vi "Fit Mutiple Cernox Files.vi"() -> ()   [LabVIEW 2025]
panel:
  out "avg T":dbl[](array[numeric])
  out "Calculated T out":dbl[][](array[numeric])
  in  "Calculate R in":dbl[](array[numeric])=[70.34796, 80.267567, 85.278681, 91.166987, 98.217159]
  out "Linear Graph":cluster{dbl[], dbl[]}[](graph)
  out "Difference":cluster{dbl[], dbl[]}[](graph)
  in  "Polynomial order":i32=18
  in  "fit mode":T1(ring)=enum."LogT-1/R"
  in  "error in":errorcluster
  in  "Sources":T2(array[cluster])=[{"File Path"=path "\\\\myhome\\NHMFLDATA/Data/PPMS/October_2025/102425/m001_164026_102425.tdms", "offset (0)"=3810, "count (-1: all)"=39060, "channel name(s) in"=["LakeShore 336 (12) A", "LakeShore 336 (12) B Raw"], "group"="p"}, {"File Path"=path "\\\\myhome\\NHMFLDATA/Data/PPMS/October_2025/102225/m003_162726_102225.tdms", "offset (0)"=134648, "count (-1: all)"=-1, "channel name(s) in"=["LakeShore 336 (12) A", "LakeShore 336 (12) B Raw"], "group"="p"}]
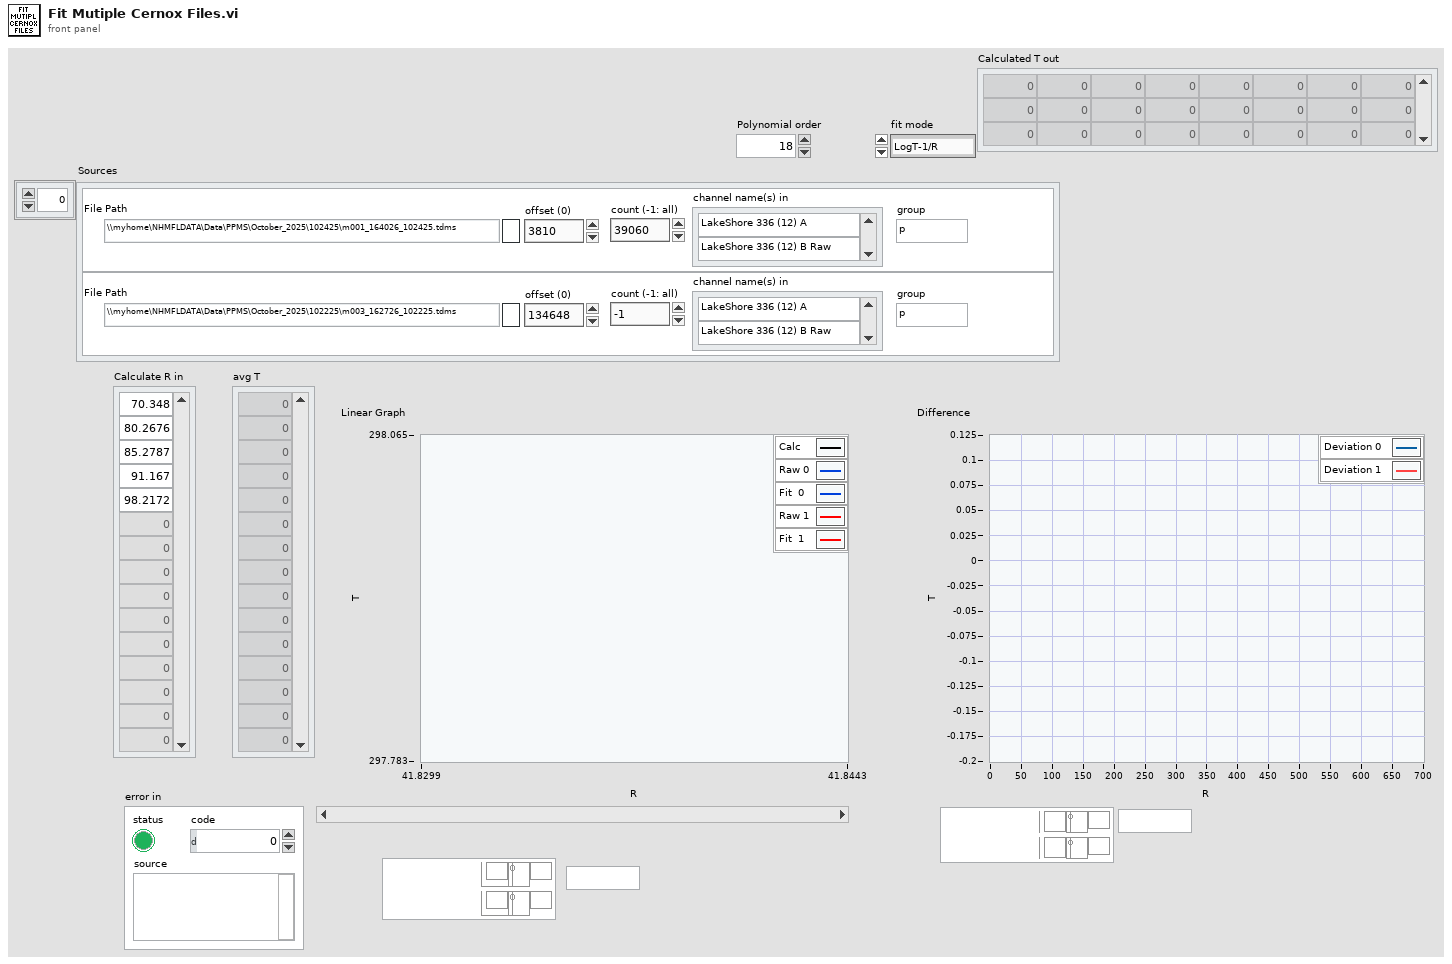
[diagram p1: front panel]
types:
  T1 = enum16{"LogT-LogR", "T-LogR", "T-R", "T-1/R", "LogT-1/R"}
  T2 = cluster{"File Path":path, "offset (0)":i64, "count (-1: all)":i64, "channel name(s) in":string[], "group":string}[]
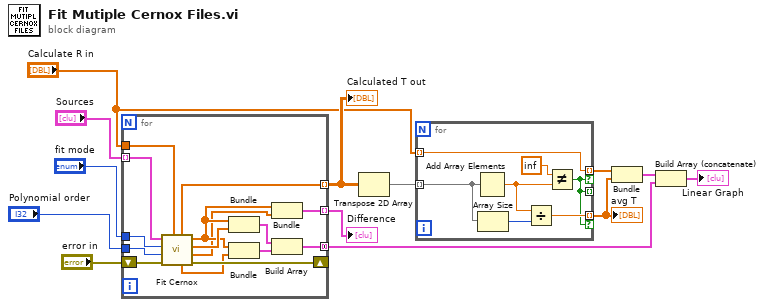
[diagram p0: block diagram]
diagram:
  n1 = for {
    tunnel: "Sources" -> [w28] mode=indexing
    shift-right: [w27] -> _
    shift-left: "error in" -> [w26]
    tunnel: "fit mode" -> [w25]
    tunnel: "Polynomial order" -> [w24]
    tunnel: [w19] -> w9 mode=concatenating
    tunnel: [w16] -> w8 mode=indexing
    tunnel: "Calculate R in" -> [w15]
    tunnel: [w14] -> w7 mode=indexing
    n2 = call "Fit Cernox.vi"("Calculate R in"=w15, "error in"=w26, "Polynomial order"=w24, "fit mode"=w25, "Raw data source"=w28) -> ("error out"=w27:errorcluster, "deviation"=w17:dbl[], "T subset"=w23:dbl[], "R"=w18:dbl[], "Fit  T"=w22:dbl[], "Calculated T out"=w14:dbl[])  [unwired: 1 in]
    n3 = Bundle("R"=w18, "T subset"=w23) -> (w21:cluster{"R":dbl[], "T subset":dbl[]})  [unwired: 1 in]
    n4 = Bundle("R"=w18, "Fit  T"=w22) -> (w20:cluster{"R":dbl[], "Fit  T":dbl[]})  [unwired: 1 in]
    n5 = Bundle("R"=w18, "deviation"=w17) -> (w16:cluster{"R":dbl[], "deviation":dbl[]})  [unwired: 1 in]
    n6 = Build Array(w21, w20) -> (w19:cluster{"R":dbl[], "Fit  T":dbl[]}[])
  }
  "Difference" <- w8
  "Calculated T out" <- w7
  n7 = Transpose 2D Array(2D array=w7) -> (transposed array=w6:dbl[][])
  n8 = for {
    tunnel: w6 -> [w34] mode=indexing
    tunnel: "Calculate R in" -> [w29] mode=indexing
    tunnel: [w32] -> w1 mode=indexing if=w31
    tunnel: [w29] -> w4 mode=indexing if=w31
    tunnel: [w31] -> _ mode=indexing
    n9 = Add Array Elements(numeric array=w34) -> (sum=w30:dbl)
    n10 = Array Size(array=w34) -> (size(s)=w33:i32)
    n11 = Divide(x=w30, y=w33) -> (x/y=w32:dbl)
    n12 = Not Equal?(x=inf, y=w30) -> (x != y?=w31:bool)
  }
  "avg T" <- w1
  n13 = Bundle(w4, w1) -> (w2:cluster{dbl[], dbl[]})  [unwired: 1 in]
  n14 = Build Array (concatenate)(w2, w9) -> (→"Linear Graph":cluster{"R":dbl[], "Fit  T":dbl[]}[])
